vi "Load_Picture.vi"(0 "Chemin In":path, 11 "error in (no error)":errorcluster caption="entrée d'erreur (pas d'erreur)") -> (4 "Img Out":picture, 6 "image data":T1, 15 "error out":errorcluster caption="sortie d'erreur")   [LabVIEW 2020, in "Library Commun.lvlib"]
uses:
  Library Commun.lvlib
  <vilib>/picture/picture.llb/imagedata.ctl
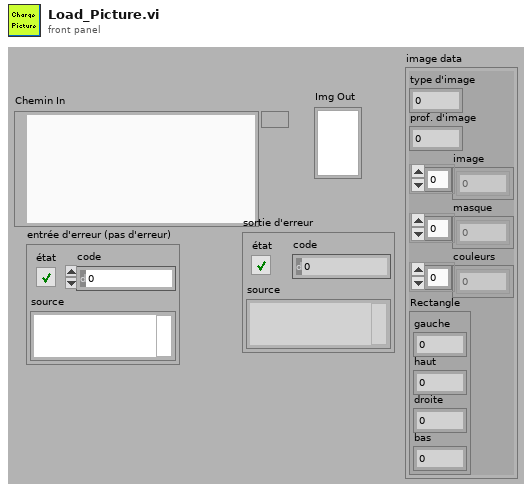
[diagram p1: front panel]
types:
  T1 = typedef "imagedata.ctl" = cluster{"image type":i32, "image depth":i32, "image":u8[], "mask":u8[], "colors":u32[], "Rectangle":cluster{"left":i16, "top":i16, "right":i16, "bottom":i16}}
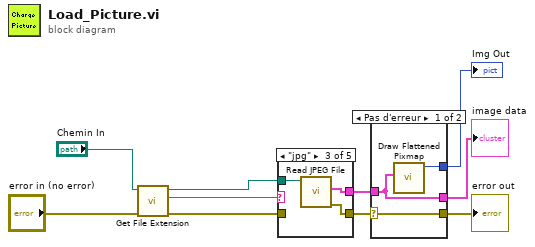
[diagram p0: block diagram]
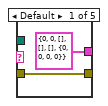
[diagram p2: hidden frame]
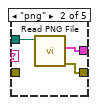
[diagram p3: hidden frame]
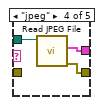
[diagram p4: hidden frame]
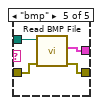
[diagram p5: hidden frame]
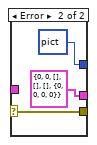
[diagram p6: hidden frame]
diagram:
  n1 = call <vilib>:"Get File Extension.vi"("error in (no error)"="error in (no error)", "file"="Chemin In") -> ("error out"=w4:errorcluster, "lowercase file extension"=w3:string, "dup file"=w5:path)  [unwired: 5 in, 2 out]
  n2 = case shown="\"jpg\"" w3 {
    tunnel: [T1 {"image type"=0, "image depth"=0, "image"=[], "mask"=[], "colors"=[], "Rectangle"={"left"=0, "top"=0, "right"=0, "bottom"=0}} ("image data") w15 w16 w19 w23] -> w10
    tunnel: w5 -> [_ w14 w18 w21 w25]
    tunnel: [w11 w13 w17 w20 w24] -> w9
    tunnel: w4 -> [w11 _ _ _ w22]
    frame Default {
    }
    frame "png" {
      n3 = call <vilib>:"Read PNG File.vi"("path to PNG file"=w14) -> ("error out"=w13:errorcluster, "image data"=w15:T1)  [unwired: 8 in, 1 out]
    }
    frame "jpg" {
      n4 = call <vilib>:"Read JPEG File.vi"("path to JPEG file"=w18) -> ("error out"=w17:errorcluster, "image data"=w16:T1)  [unwired: 8 in, 1 out]
    }
    frame "jpeg" {
      n5 = call <vilib>:"Read JPEG File.vi"("path to JPEG file"=w21) -> ("error out"=w20:errorcluster, "image data"=w19:T1)  [unwired: 8 in, 1 out]
    }
    frame "bmp" {
      n6 = call <vilib>:"Read BMP File.vi"("error in (no error)"=w22, "path to BMP file"=w25) -> ("error out"=w24:errorcluster, "image data"=w23:T1)  [unwired: 7 in, 1 out]
    }
  }
  n7 = case shown="Pas d'erreur" w9 {
    selector: w9 -> [w26 w29]
    tunnel: w10 -> [w27 _]
    tunnel: [w28 picture data[5B] ("Img Out")] -> w8
    tunnel: [w27 T1 {"image type"=0, "image depth"=0, "image"=[], "mask"=[], "colors"=[], "Rectangle"={"left"=0, "top"=0, "right"=0, "bottom"=0}} ("image data")] -> w7
    tunnel: [w26 w29] -> w1
    frame No Error {
      n8 = call <vilib>:"Draw Flattened Pixmap.vi"("image data"=w27) -> ("new picture"=w28:picture)  [unwired: 1 in, 7 out]
    }
    frame Error {
    }
  }
  "Img Out" <- w8
  "image data" <- w7
  "error out" <- w1
